vi "Write Element of Array of ccd.vi"(8 "error in (no error)":errorcluster, 9 "Hardware.lvlib:CCD.lvlib:CCD.lvclass":refnum<class "CCD.lvclass">, 10 "index":i32, 11 "CCD monitor in":refnum<class "CCD monitor.lvclass">) -> (0 "error out":errorcluster, 3 "CCD monitor out":refnum<class "CCD monitor.lvclass">)   [LabVIEW 2016, in "Hardware.lvlib" / "CCD monitor.lvlib" / "CCD monitor.lvclass"]
uses:
  <userlib>/Common Components/Hardware/Abstract System/Monitor/CCD monitor.lvclass
  <userlib>/Common Components/Hardware/CCD/CCD/CCD.lvclass
  <userlib>/Common Components/Hardware/Abstract System/Monitor/CCD monitor.lvclass/CCD monitor.ctl
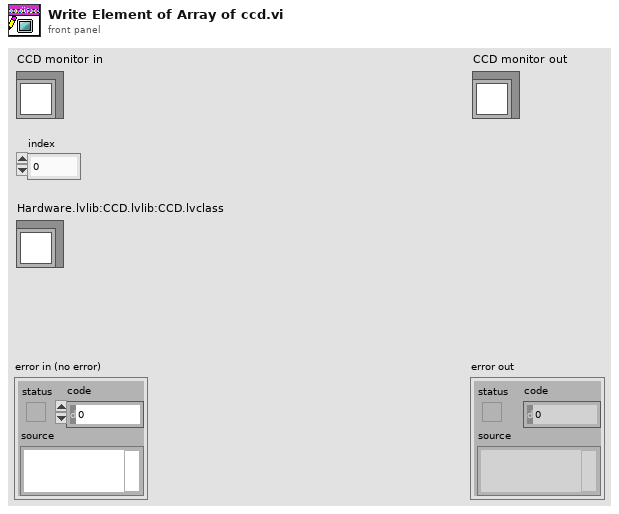
[diagram p1: front panel]
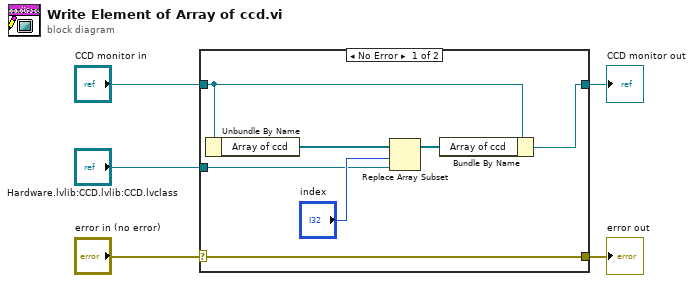
[diagram p0: block diagram]
diagram:
  n1 = case shown="No Error" "error in (no error)" {
    selector: "error in (no error)" -> [w12 w13]
    tunnel: [w12 w13] -> w4
    tunnel: [w11 w14] -> w2
    tunnel: "CCD monitor in" -> [w10 w14]
    tunnel: "Hardware.lvlib:CCD.lvlib:CCD.lvclass" -> [w6 _]
    frame No Error {
      n2 = Unbundle By Name(w10) -> ("Array of ccd"=w9:refnum<class "CCD.lvclass">[])
      n3 = Replace Array Subset(array=w9, new element=w6, index="index") -> (w8:refnum<class "CCD.lvclass">[])
      n4 = Bundle By Name(cluster=w10, "Array of ccd"=w8) -> (w11:refnum<class "CCD monitor.lvclass">)
    }
    frame Error {
    }
  }
  "error out" <- w4
  "CCD monitor out" <- w2
